vi "Configure Remote Trace Destination.vi"(8 "error in (no error)":errorcluster, 9 "File Name (\"RemoteTrace.log\")":string="RemoteTrace.log", 10 "Target (File)":i32(ring)=1 items=["Screen", "File", "Screen and file"], 11 "VISA resource name":refnum<visa-resource-name>) -> (0 "error out":errorcluster, 3 "VISA resource name out":refnum<visa-resource-name>)   [LabVIEW 2015, in "Rohde&Schwarz CMXP Base.lvlib"]
doc: "Selects the trace log destination. You can display the log in the GUI and/or write the results to a file.\n\nAttribute:\n-\n\nRemote-control command:\n[CONFigure:]BASE:RTRace:TARGet"
uses:
  <instrlib>/Rohde&Schwarz CMXP Base/Rohde&Schwarz CMXP Base.lvlib
  <instrlib>/Rohde&Schwarz CMXP Base/Private/rsidr_core.llb/rsidr_core.lvlib
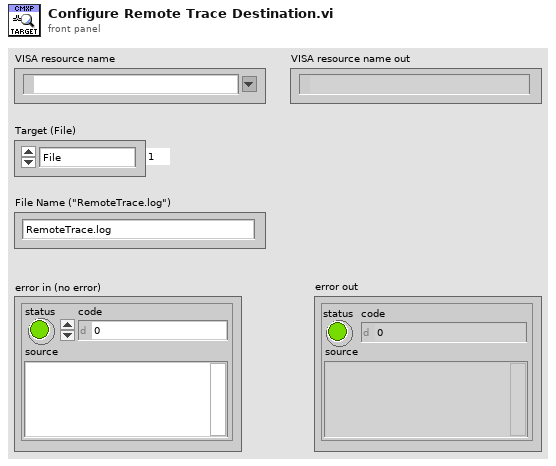
[diagram p1: front panel]
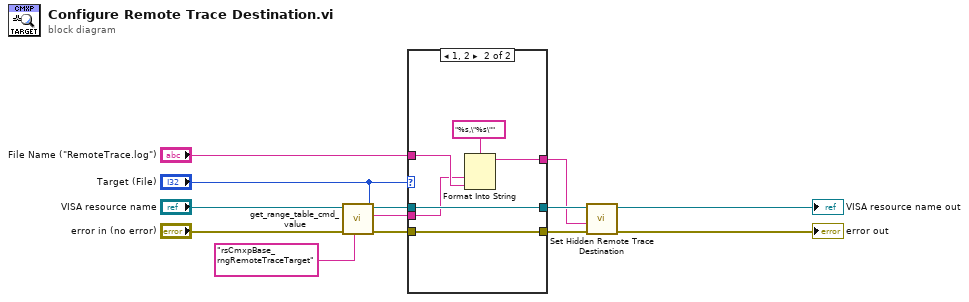
[diagram p0: block diagram]
diagram:
  n1 = call <instrlib>:"get_range_table_cmd_value.vi"("Range Table ID in"="rsCmxpBase_rngRemoteTraceTarget", "error in"="error in (no error)", "Input Int32 value"="Target (File)", "VISA resource name"="VISA resource name") -> ("error out"=w10:errorcluster, "Cmd value out"=w6:string, "VISA resource name out"=w3:refnum<visa-resource-name>)  [unwired: 5 in]
  n2 = case shown="1, 2" "Target (File)" {
    tunnel: w10 -> [w16 w19]
    tunnel: [w16 w19] -> w9
    tunnel: [w14 w22] -> w1
    tunnel: w6 -> [w14 w17]
    tunnel: "File Name (\"RemoteTrace.log\")" -> [_ w18]
    tunnel: w3 -> [w15 w20]
    tunnel: [w15 w20] -> w2
    frame Default {
    }
    frame 1, 2 {
      n3 = Format Into String(format string="%s,\"%s\"", w17, w18) -> (resulting string=w22:string)  [unwired: 2 in, 1 out]
    }
  }
  n4 = call "Set Hidden Remote Trace Destination"("error in (no error)"=w9, "Hidden Remote Trace Destination ()"=w1, "instrument handle"=w2) -> ("error out"=→"error out":errorcluster, "instrument handle out"=→"VISA resource name out":refnum<visa-resource-name>)  [unwired: 7 in]
